vi ".NET Object to GObject.vi"(8 "error in (no error)":errorcluster, 10 ".NET Object":refnum<k24>) -> (0 "error out":errorcluster, 2 "G Object":variant)   [LabVIEW 2018, in "G .NET.lvlib"]
uses:
  G .NET.lvlib
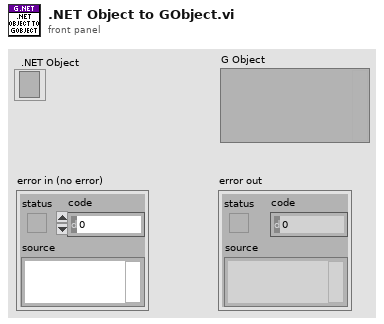
[diagram p1: front panel]
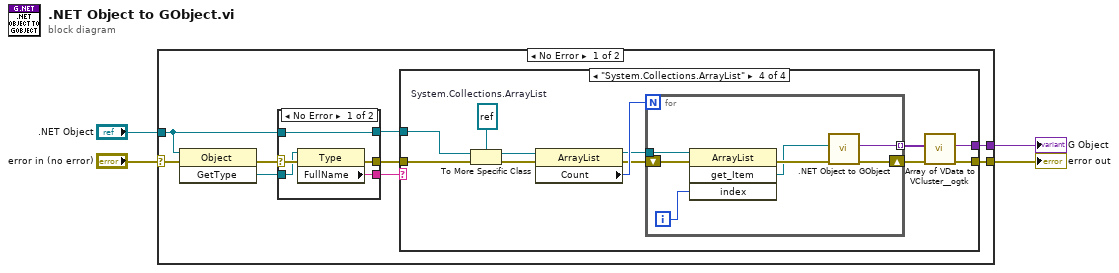
[diagram p0: block diagram]
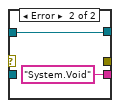
[diagram p2: hidden frame]
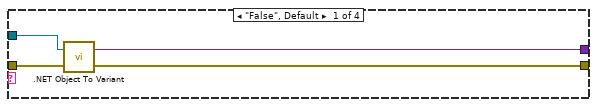
[diagram p3: hidden frame]
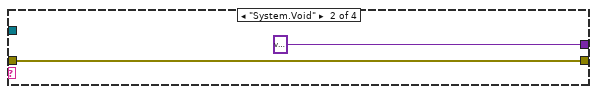
[diagram p4: hidden frame]
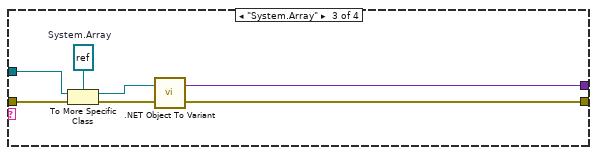
[diagram p5: hidden frame]
diagram:
  n1 = case shown="No Error" "error in (no error)" {
    selector: "error in (no error)" -> [w13 w53]
    tunnel: [w12 w53] -> w3
    tunnel: ".NET Object" -> [w9 _]
    tunnel: [w11 _] -> w1
    frame No Error {
      n2 = invoke class="Object" method="GetType"(reference=w9, error in=w13) -> (error out=w10:errorcluster, "GetType"=w6:refnum<k24>)  [unwired: 1 in, 1 out]
      n3 = case shown="No Error" w10 {
        selector: w10 -> [w16 _]
        tunnel: w6 -> [w15 _]
        tunnel: [w18 _] -> w8
        tunnel: [w17 "System.Void"] -> w7
        tunnel: w9 -> [w14 w19]
        tunnel: [w14 w19] -> w5
        frame No Error {
          n4 = property class="Type"(reference=w15, error in=w16) -> (error out=w18:errorcluster, "FullName"=w17:string)  [unwired: 1 out]
        }
        frame Error {
        }
      }
      n5 = case shown="\"System.Collections.ArrayList\"" w7 {
        tunnel: w5 -> [w23 _ w32 w45]
        tunnel: w8 -> [w24 w26 w33 w44]
        tunnel: [w21 w26 w28 w35] -> w12
        tunnel: [w22 variant ("Void") w27 w34] -> w11
        frame "False", Default {
          n6 = call <vilib>:".NET Object To Variant.vi"("error in (no error)"=w24, ".NET object"=w23) -> ("error out"=w21:errorcluster, "variant"=w22:variant)
        }
        frame "System.Void" {
        }
        frame "System.Array" {
          w31 = refnum<k24> refnum  # System.Array
          n7 = To More Specific Class(target class=w31, reference=w32, error in=w33) -> (specific class reference=w29:refnum<k24>, error out=w30:errorcluster)
          n8 = call <vilib>:".NET Object To Variant.vi"("error in (no error)"=w30, ".NET object"=w29) -> ("error out"=w28:errorcluster, "variant"=w27:variant)
        }
        frame "System.Collections.ArrayList" {
          w43 = refnum<k24> refnum  # System.Collections.ArrayList
          n9 = To More Specific Class(target class=w43, reference=w45, error in=w44) -> (specific class reference=w42:refnum<k24>, error out=w41:errorcluster)
          n10 = property class="ArrayList"(reference=w42, error in=w41) -> (reference out=w38:refnum<k24>, error out=w39:errorcluster, "Count"=w40:i32)
          n11 = for {
            N: w40 -> [_]
            shift-right: [w48] -> w37
            shift-left: w39 -> [w51]
            tunnel: w38 -> [w50]
            tunnel: [w49] -> w36 mode=indexing
            i -> [w52]
            n12 = invoke class="ArrayList" method="get_Item"(reference=w50, error in=w51, "index"=w52) -> (error out=w47:errorcluster, "get_Item"=w46:refnum<k24>)  [unwired: 1 in, 2 out]
            n13 = call ".NET Object to GObject.vi"("error in (no error)"=w47, ".NET Object"=w46) -> ("error out"=w48:errorcluster, "G Object"=w49:variant)  [unwired: 8 in]
          }
          n14 = call <userlib>:"Array of VData to VCluster__ogtk.vi"("error in (no error)"=w37, "Array"=w36) -> ("error out"=w35:errorcluster, "VCluster"=w34:variant)  [unwired: 8 in]
        }
      }
    }
    frame Error {
    }
  }
  "error out" <- w3
  "G Object" <- w1
